vi "setUp.vi"(8 "error in (no error)":errorcluster, 11 "reference in":refnum<class "suite SSL Client.lvclass">) -> (0 "error out":errorcluster, 3 "reference out":refnum<class "suite SSL Client.lvclass">)   [LabVIEW 2013, in "suite SSL Client.lvclass"]
doc: "setUp runs prior to the test method during test execution. Use this method to initialize any object data required by your tests."
uses:
  suite SSL Client.lvclass
  <vilib>/addons/_JKI Toolkits/VI Tester/TestSuite.llb/TestSuite.lvclass
  SSL_Lib/SSL-Lib/SSL-Lib.lvclass
  SSL_Lib/SSL-Lib/Library Paths.ctl
  SSL Context.vi
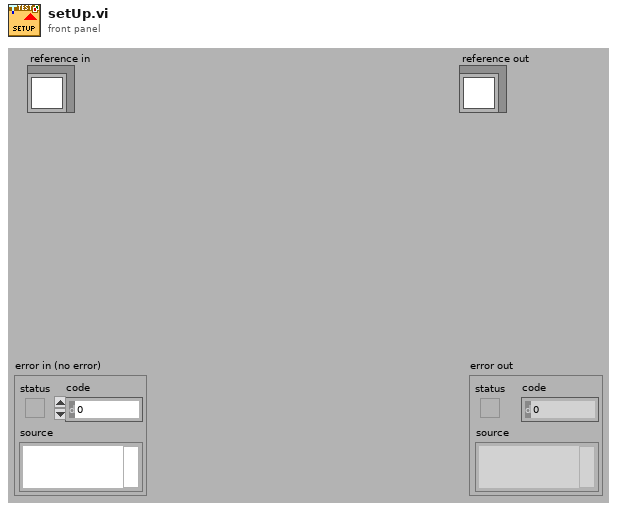
[diagram p1: front panel]
types:
  T1 = typedef "SSL_Lib.lvlib/SSL-Lib.lvclass/Library Paths.ctl" = cluster{"SSL Library Path":path, "Crypto Library Path":path}
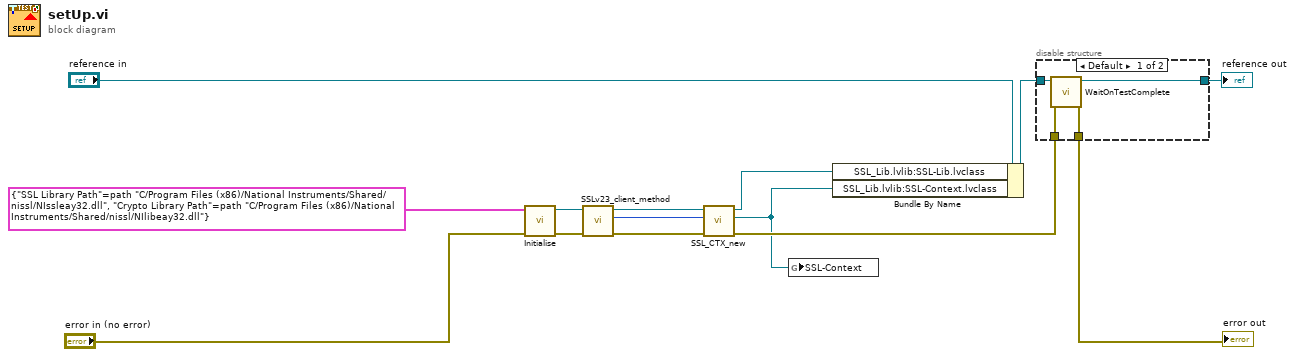
[diagram p0: block diagram]
diagram:
  n1 = call "Initialise.vi"("error in (no error)"="error in (no error)", "Library Paths"=T1 {"SSL Library Path"=path "C:/Program Files (x86)/National Instruments/Shared/nissl/NIssleay32.dll", "Crypto Library Path"=path "C:/Program Files (x86)/National Instruments/Shared/nissl/NIlibeay32.dll"}) -> ("error out"=w7:errorcluster, "SSL-Lib out"=w10:refnum<class "SSL-Lib.lvclass">)  [unwired: 8 in]
  n2 = call "SSLv23_client_method.vi"("error in (no error)"=w7, "SSL-Lib in"=w10) -> ("error out"=w6:errorcluster, "*SSL_Method"=w9:u64, "SSL-Lib out"=w8:refnum<class "SSL-Lib.lvclass">)  [unwired: 7 in]
  n3 = call "SSL_CTX_new.vi"("error in (no error)"=w6, "*SSL_Method"=w9, "SSL-Lib in"=w8) -> ("error out"=w3:errorcluster, "SSL-Context out"=w1:refnum<class "SSL-Context.lvclass">, "SSL-Lib out"=w2:refnum<class "SSL-Lib.lvclass">)  [unwired: 6 in]
  n4 = global write "SSL Context.vi" "SSL-Context"(w1) -> ()
  n5 = Bundle By Name(cluster="reference in", "SSL_Lib.lvlib:SSL-Lib.lvclass"=w2, "SSL_Lib.lvlib:SSL-Context.lvclass"=w1) -> (w13:refnum<class "suite SSL Client.lvclass">)
  n6 = disable-structure shown="Default" {
    disable-tunnel: w13 -> [w18 w19]
    disable-tunnel: [w17 w19] -> w12
    disable-tunnel: w3 -> [w16 w20]
    disable-tunnel: [w15 w20] -> w11
    frame condition #0 (active) {
      n7 = call <vilib>:"WaitOnTestComplete.vi"("error in (no error)"=w16, "TestSuite in"=w18) -> ("error out"=w15:errorcluster, "TestSuite out"=w17:refnum<class "suite SSL Client.lvclass">)  [unwired: 8 in]
    }
    frame condition #1 {
    }
  }
  "error out" <- w11
  "reference out" <- w12
